vi "Get Redirection URL (HTTP 302).vi"(8 "error in (no error)":errorcluster, 11 "HTTP GET Header":string) -> (0 "error out":errorcluster, 1 "redirection":bool, 3 "Redirection URL":string)   [LabVIEW 2021, in "Web.lvlib"]
uses:
  Web.lvlib
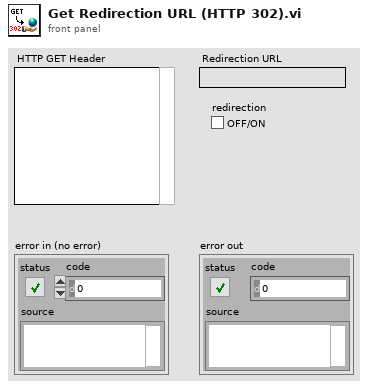
[diagram p1: front panel]
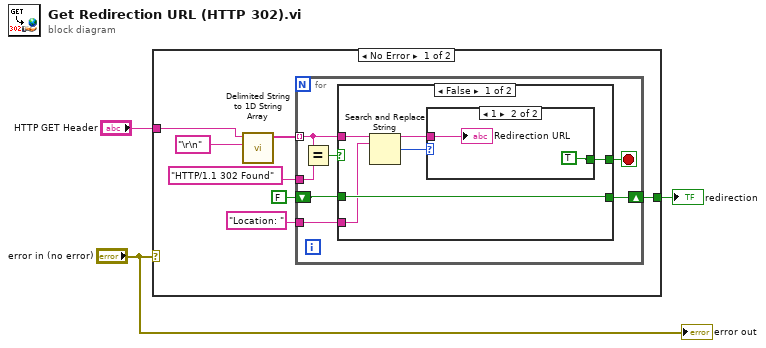
[diagram p0: block diagram]
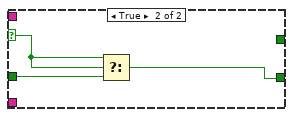
[diagram p3: hidden frame]
diagram:
  n1 = case shown="No Error" "error in (no error)" {
    tunnel: "HTTP GET Header" -> [w10 _]
    tunnel: [w5 _] -> w2
    frame No Error {
      n2 = call <vilib>:"Delimited String to 1D String Array.vi"("delimiter"="\r\n", "delimited string"=w10) -> ("string array"=w8:string[])  [unwired: 9 in]
      n3 = for {
        tunnel: w8 -> [w13] mode=indexing
        tunnel: "HTTP/1.1 302 Found" ("search string") -> [w17]
        shift-right: [w14] -> w5
        shift-left: FALSE -> [w15]
        tunnel: "Location: " ("search string") -> [w12]
        stop <- w11 stop-if-true
        n4 = Equal?(x=w13, y=w17) -> (x = y?=w16:bool)
        n5 = case shown="False" w16 {
          selector: w16 -> [_ w28]
          tunnel: w15 -> [w23 w27]
          tunnel: [w23 w26] -> w14
          tunnel: w13 -> [w22 _]
          tunnel: w12 -> [w21 _]
          tunnel: [w18 _] -> w11
          frame False {
            n6 = Search and Replace String(input string=w22, search string=w21) -> (result string=w19:string, number of replacements=w20:i32)  [unwired: 6 in, 2 out]
            n7 = case shown="1" w20 {
              tunnel: w19 -> [_ w25]
              tunnel: [_ TRUE] -> w18
              frame 0, Default {
              }
              frame 1 {
                "Redirection URL" <- w25
              }
            }
          }
          frame True {
            n8 = Select(t=w28, s=w28, f=w27) -> (s? t:f=w26:bool)
          }
        }
      }
    }
    frame Error {
    }
  }
  "redirection" <- w2
  "error out" <- "error in (no error)"
